vi "Return_Gauge_FS_SubVi.vi"(10 "number":dbl, 11 "Knob in":refnum<vi>) -> (3 "Gauge":dbl(knob) scale=0.0..100.0)   [LabVIEW 2014]
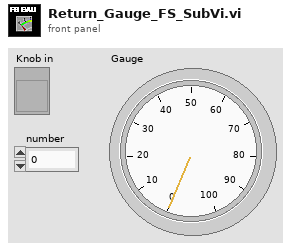
[diagram p1: front panel]
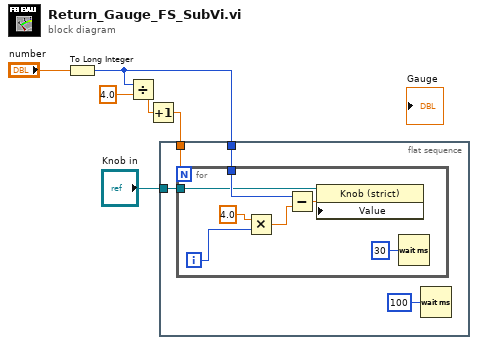
[diagram p0: block diagram]
diagram:
  n1 = To Long Integer(number="number") -> (32bit integer=w1:i32)
  n2 = Divide(x=w1, y=4.0) -> (x/y=w5:dbl)
  n3 = Increment(x=w5) -> (x+1=w6:dbl)
  n4 = flat-sequence {
    tunnel: w6 -> [w9]
    tunnel: w1 -> [w8]
    tunnel: "Knob in" -> [w7]
    frame #0 {
      n5 = for {
        N: w9 -> [_]
        tunnel: w8 -> [w13]
        tunnel: w7 -> [w11]
        i -> [w15]
        n6 = Multiply(x=4.0, y=w15) -> (x*y=w16:dbl)
        n7 = Subtract(x=w13, y=w16) -> (x-y=w12:dbl)
        n8 = property class="Knob (strict)"(reference=w11, "Value"=w12) -> ()  [unwired: 1 in, 2 out]
        n9 = Wait (ms)(milliseconds to wait=u32 30) -> ()  [unwired: 1 out]
      }
      n10 = Wait (ms)(milliseconds to wait=u32 100) -> ()  [unwired: 1 out]
    }
  }
